vi "Get Workbook.vi"(8 "error in (no error)":errorcluster, 11 "Excel Legacy in":refnum<class "Excel Legacy.lvclass">) -> (0 "error out":errorcluster, 2 "Workbook":refnum<k24>, 3 "Excel Legacy out":refnum<class "Excel Legacy.lvclass">)   [LabVIEW 2013, in "Excel Legacy.lvclass"]
uses:
  Excel Legacy.lvclass
  C:/PhaeronGit/LVNPOI/Resources/NPOI 2.1.1 dotnet2/NPOI.dll
  Resources/NPOI 2.1.1 dotnet2/NPOI.dll
  Excel Legacy.lvclass/Excel Legacy.ctl
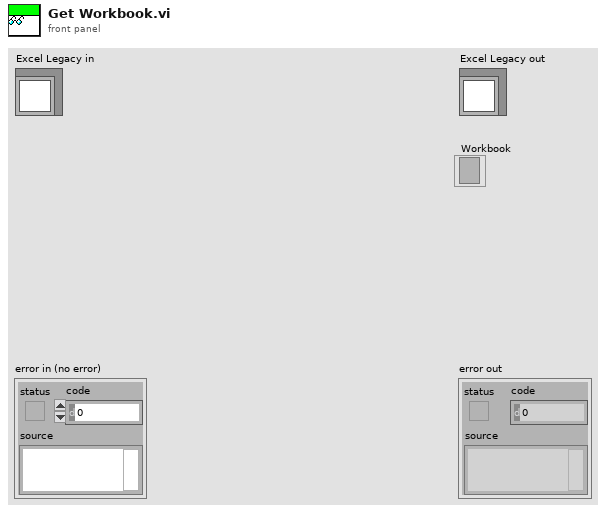
[diagram p1: front panel]
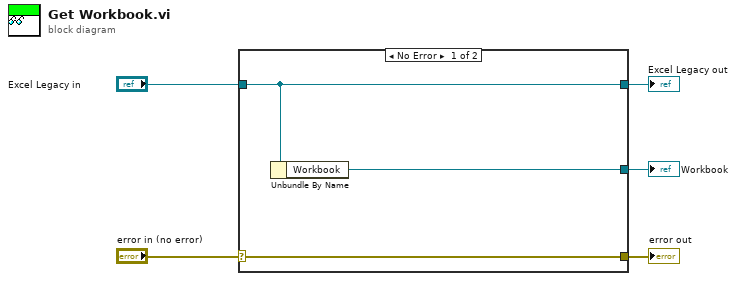
[diagram p0: block diagram]
diagram:
  n1 = case shown="No Error" "error in (no error)" {
    selector: "error in (no error)" -> [w8 w9]
    tunnel: [w8 w9] -> w4
    tunnel: [w7 w10] -> w2
    tunnel: "Excel Legacy in" -> [w7 w10]
    tunnel: [w6 _] -> w1
    frame No Error {
      n2 = Unbundle By Name(w7) -> ("Workbook"=w6:refnum<k24>)
    }
    frame Error {
    }
  }
  "error out" <- w4
  "Excel Legacy out" <- w2
  "Workbook" <- w1
